vi "_FPGA_Accumulator_U64.vi"(6 "Reset_latch":bool, 8 "shift_in":u64, 10 "Increment_in":u64) -> (1 "Next_Accumalated_U64_out":u64, 2 "Accumulated_U64_out":u64)   [LabVIEW 2018]
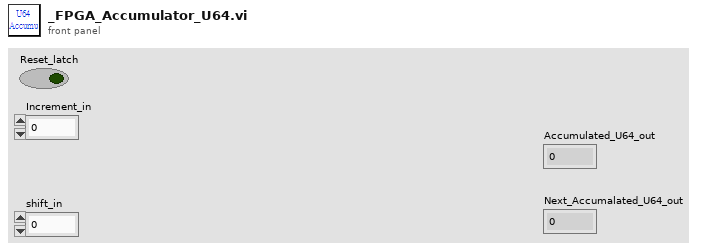
[diagram p1: front panel]
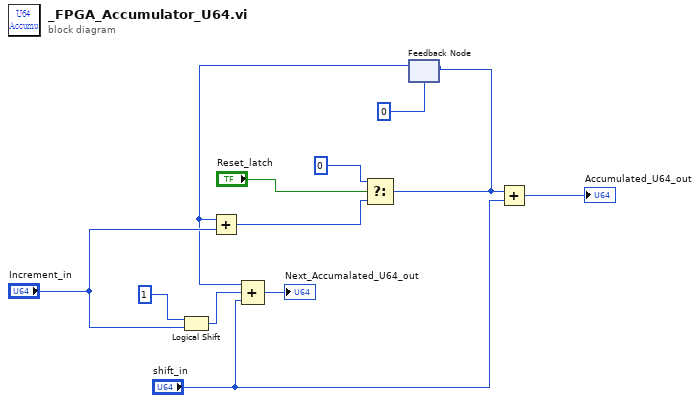
[diagram p0: block diagram]
diagram:
  n1 = Logical Shift(y=i16 1, x="Increment_in") -> (x << y=w3:u64)
  n2 = feedback #1(u64 0 ("t")) -> (w5:u64)
  n3 = Add(x=w5, y="Increment_in") -> (x+y=w6:u64)
  n4 = Compound Arithmetic op=ADD(w5, w3, "shift_in") -> (→"Next_Accumalated_U64_out":u64)
  n5 = Select(t=u64 0, s="Reset_latch", f=w6) -> (s? t:f=w8:u64)
  n6 = feedback-in #1(w8) -> ()
  n7 = Add(x=w8, y="shift_in") -> (x+y=→"Accumulated_U64_out":u64)
